vi "Determine Sides.vi"(8 "error in (no error)":errorcluster, 11 "Tile in":refnum<class "Tile.lvclass">) -> (0 "error out":errorcluster, 3 "Tile out":refnum<class "Tile.lvclass">)   [LabVIEW 2020, in "Tile.lvclass"]
uses:
  Tile.lvclass
  Tile.lvclass/Tile.ctl
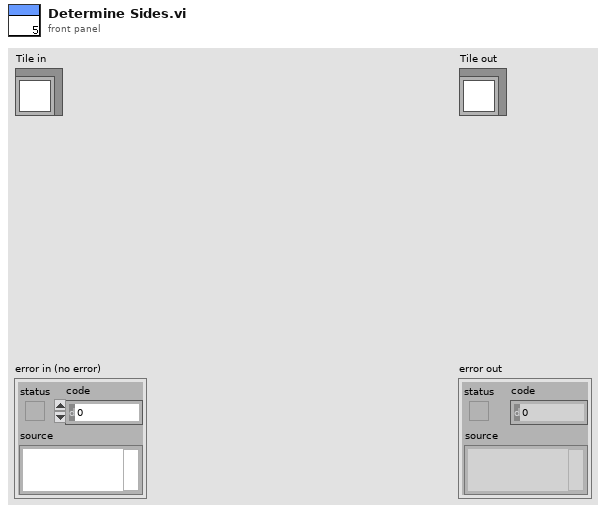
[diagram p1: front panel]
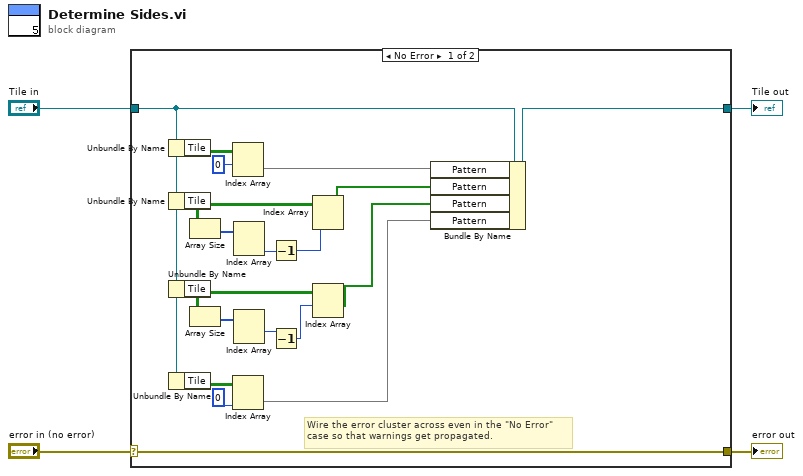
[diagram p0: block diagram]
diagram:
  n1 = case shown="No Error" "error in (no error)" {
    selector: "error in (no error)" -> [w23 w25]
    tunnel: [w23 w25] -> w3
    tunnel: [w6 w24] -> w1
    tunnel: "Tile in" -> [w5 w24]
    frame No Error {
      # "Wire the error cluster across even in the \"No Error\"\ncase so that warnings get propagated."
      n2 = Unbundle By Name(w5) -> ("Tile"=w22:bool[][])
      n3 = Unbundle By Name(w5) -> ("Tile"=w20:bool[][])
      n4 = Unbundle By Name(w5) -> ("Tile"=w15:bool[][])
      n5 = Unbundle By Name(w5) -> ("Tile"=w12:bool[][])
      n6 = Array Size(array=w20) -> (size(s)=w19:i32[])
      n7 = Array Size(array=w15) -> (size(s)=w16:i32[])
      n8 = Index Array(array=w22, index (row)=0) -> (element=w10:bool[])  [unwired: 1 in]
      n9 = Index Array(array=w12, index (col)=0 ("index (row)")) -> (element=w7:bool[])  [unwired: 1 in]
      n10 = Index Array(array=w19) -> (element #2=w18:i32)  [unwired: 2 in, 1 out]
      n11 = Index Array(array=w16) -> (element #1=w14:i32)  [unwired: 2 in, 1 out]
      n12 = Decrement(x=w18) -> (x-1=w17:i32)
      n13 = Decrement(x=w14) -> (x-1=w13:i32)
      n14 = Index Array(array=w20, index (col)=w17) -> (element=w9:bool[])  [unwired: 1 in]
      n15 = Index Array(array=w15, index (row)=w13) -> (element=w8:bool[])  [unwired: 1 in]
      n16 = Bundle By Name(cluster=w5, "Pattern"=w10, "Pattern"=w9, "Pattern"=w8, "Pattern"=w7) -> (w6:refnum<class "Tile.lvclass">)
    }
    frame Error {
    }
  }
  "error out" <- w3
  "Tile out" <- w1
